vi "move_to_angle.vi"(6 "proportional":sgl=0.5 format="%#_13g", 9 "Port (All Ports)入力":T1 items=["Port A"=0, "Port B"=1, "Port C"=2, "Ports A & B"=4, "Ports A & C"=5, "Ports B & C"=6, "All Ports"=3], 10 "desired position":i32=320, 11 "Di":sgl=0.05 format="%#_13g") -> ()   [LabVIEW 2016, in "main.lvrbt"]
uses:
  main.lvrbt
  <vilib>/NXT/Subs/MotorOutput.ctl
  <vilib>/NXT/Dual Mode Library/Motors/ResetMotor.vi
  <vilib>/NXT/Dual Mode Library/Motors/Rotation.vi
  <vilib>/NXT/Dual Mode Library/Motors/MotorOn.vi
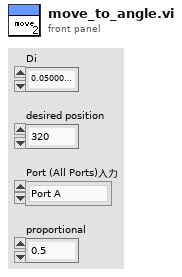
[diagram p1: front panel]
types:
  T1 = typedef "MotorOutput.ctl" = u8
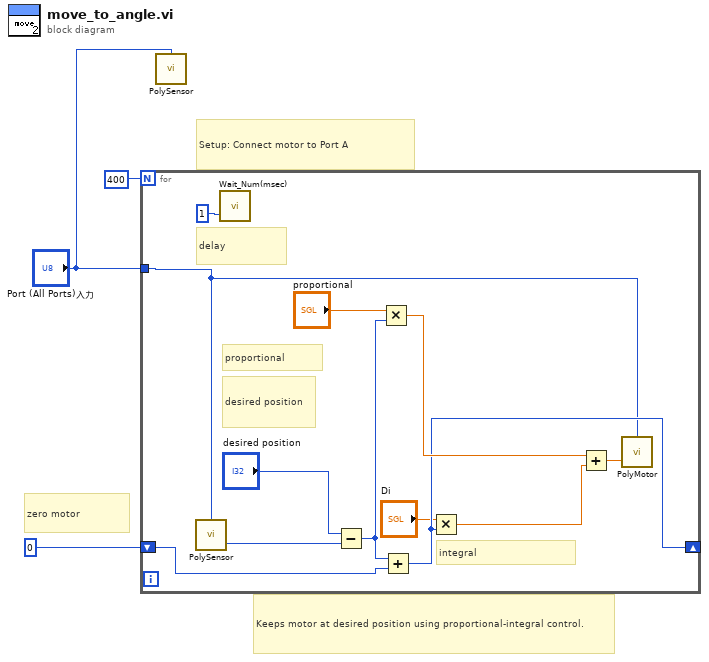
[diagram p0: block diagram]
diagram:
  # "zero motor"
  # "Keeps motor at desired position using proportional-integral control."
  # "Setup: Connect motor to Port A"
  n1 = for {
    N: 400 -> [_]
    shift-right: [w10] -> _
    shift-left: 0 ("RotationCount") -> [w14]
    tunnel: "Port (All Ports)入力" -> [w4]
    # "integral"
    # "proportional"
    # "desired position"
    # "delay"
    n2 = call-poly <vilib>:"PolySensor.vi"("Port (Port A)"=w4) -> ("Angle of Rotation"=w7:i32)  [unwired: 1 in, 2 out]
    n3 = call <vilib>:"Wait_Num(msec).vi"("Time (100 msec)"=u32 1 ("milliseconds to wait")) -> ()  [unwired: 3 in, 1 out]
    n4 = Subtract(x="desired position", y=w7) -> (x-y=w11:i32)
    n5 = Multiply(x="proportional", y=w11) -> (x*y=w13:sgl)
    n6 = Add(x=w11, y=w14) -> (x+y=w10:i32)
    n7 = Multiply(x="Di", y=w10) -> (x*y=w8:sgl)
    n8 = Add(x=w13, y=w8) -> (x+y=w6:sgl)
    n9 = call-poly <vilib>:"PolyMotor.vi"("Power (75)"=w6, "Output Port (All Ports)"=w4) -> ()  [unwired: 1 in, 2 out]
  }
  n10 = call-poly <vilib>:"PolySensor.vi"("Port (All Ports)"="Port (All Ports)入力") -> ()  [unwired: 1 in, 3 out]
